vi "Processing the actuator action without wait for Running Signal.vi"(7 "error in (no error)":errorcluster, 8 "Actuator Name":string, 9 "Time to wait":i32=999, 10 "UTP IO Session in":T1) -> ()   [LabVIEW 2023, in "Actuators.lvlib"]
doc: "Processing actutor action\nPeriod for reading is 10ms"
uses:
  Actuators.lvlib
  <vilib>/Noffz/UTP IO/UTP IO Library/Typedefs/Session Handle.ctl
  <vilib>/Noffz/UTP IO/UTP IO Library/UTP IO Pool Session.lvclass
  f0ffdedf-838d-4681-b715-cdd8ad4b0fb5.vi
  <vilib>/Noffz/UTP IO/UTP IO Library/methods/poly/plc/Write PLC Variable (Boolean).vi
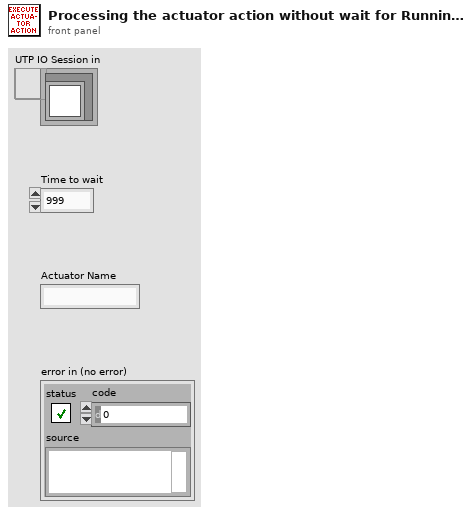
[diagram p1: front panel]
types:
  T1 = typedef "UTP IO Library.lvlib/UTP IO Pool Session.lvclass/Session Handle.ctl" = refnum<data-value>
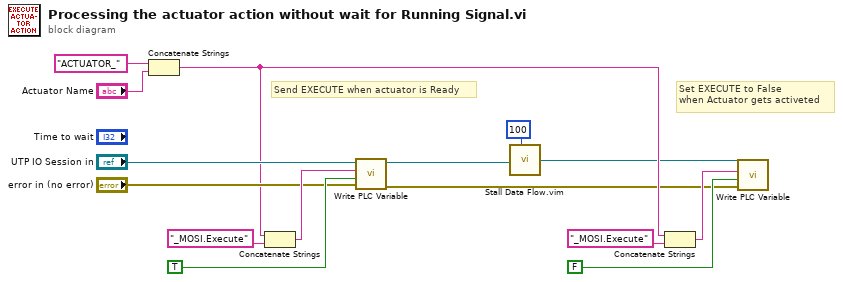
[diagram p0: block diagram]
diagram:
  # "Set EXECUTE to False \nwhen Actuator gets activeted"
  # "Send EXECUTE when actuator is Ready"
  n1 = Concatenate Strings("ACTUATOR_" ("string"), "Actuator Name") -> (w6:string)
  n2 = Concatenate Strings(w6, "_MOSI.Execute" ("string")) -> (w15:string)
  n3 = call-poly <vilib>:"Write PLC Variable.vi"("error in (no error)"="error in (no error)", "value"=TRUE, "variable name"=w15, "UTP IO Session in"="UTP IO Session in") -> ("error out"=w2:errorcluster, "UTP IO Session out"=w4:T1)  [unwired: 6 in]
  n4 = call "Stall Data Flow.vim"("value in"=w4, "milliseconds to wait"=u32 100) -> ("value out"=w3:T1)  [unwired: 1 out]
  n5 = Concatenate Strings(w6, "_MOSI.Execute" ("string")) -> (w11:string)
  n6 = call-poly <vilib>:"Write PLC Variable.vi"("error in (no error)"=w2, "value"=FALSE, "variable name"=w11, "UTP IO Session in"=w3) -> ()  [unwired: 6 in, 2 out]
